vi "ConfigureTrigSource.vi"(8 "error in (no error)":errorcluster, 11 "Instrument Handle":refnum<k15>) -> (0 "error out":errorcluster, 3 "Instrument Handle Out":refnum<k15>)   [LabVIEW 2020]
uses:
  <instrlib>/niFgen/niFgen.llb/niFgen_ctl Trigger Source Values (Ring).ctl
  <instrlib>/niFgen/niFgen.llb/niFgen_ctl Trigger DigEdge - Edge Values (Ring).ctl
  <instrlib>/niFgen/niFgen.llb/niFgen Configure Digital Edge Start Trigger.vi
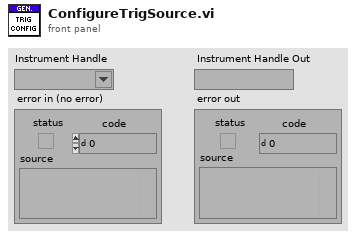
[diagram p1: front panel]
types:
  T1 = typedef "niFgen_ctl Trigger DigEdge - Edge Values (Ring).ctl" = i32
  T2 = typedef "niFgen_ctl Trigger Source Values (Ring).ctl" = string
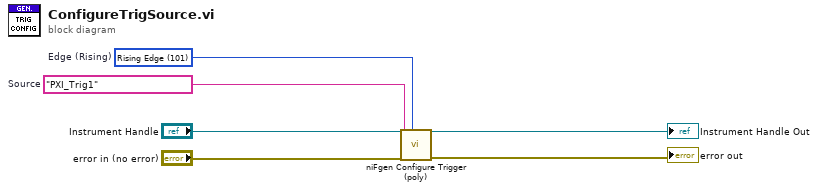
[diagram p0: block diagram]
diagram:
  w3 = T1 101 items=["Rising Edge"=101, "Falling Edge"=102]  # Edge (Rising)
  w4 = T2 "PXI_Trig1"  # Source
  n1 = call-poly <instrlib>:"niFgen Configure Trigger (poly).vi"("Edge (Rising)"=w3, "error in (no error)"="error in (no error)", "Source"=w4, "Instrument Handle"="Instrument Handle") -> ("error out"=→"error out":errorcluster, "Instrument Handle Out"=→"Instrument Handle Out":refnum<k15>)  [unwired: 6 in]
